vi "read_config.vi"() -> ()   [LabVIEW 2015]
uses:
  <vilib>/Utility/config.llb/Read Key (String).vi
  global/tcp_conn.vi
  global_config.vi
  <vilib>/Utility/config.llb/NI_LVConfig.lvlib
panel:
  out "服务器IP地址":string
  out "配置信息输出":T1
  out "默认上传数据输出":string[](array[string])
  out "value":string caption="data"
  out "info":string[](array[string])
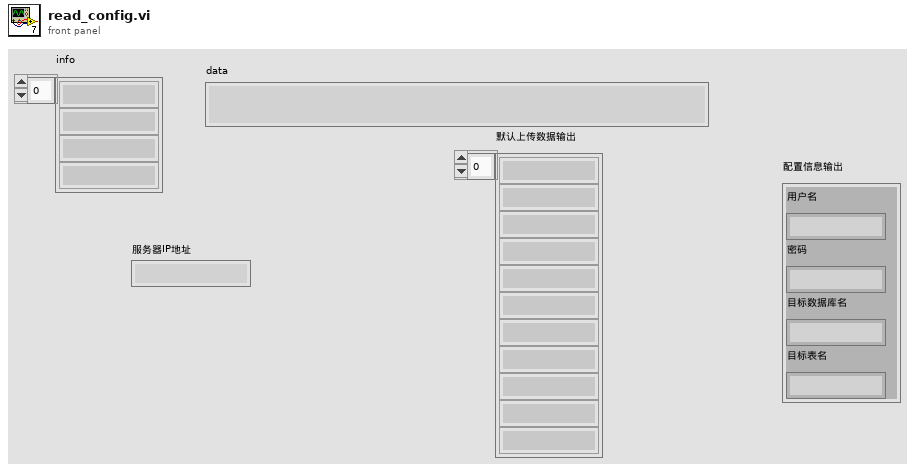
[diagram p1: front panel]
types:
  T1 = cluster{"用户名":string, "密码":string, "目标数据库名":string, "目标表名":string}
  T2 = enum32{"invalid app kind", "Development System", "Run Time System", "Student Edition", "Embedded LabVIEW", "Evaluation", "Custom"}
  T3 = typedef "NI_LVConfig.lvlib/Config Data RefNum.ctl" = refnum<k1>
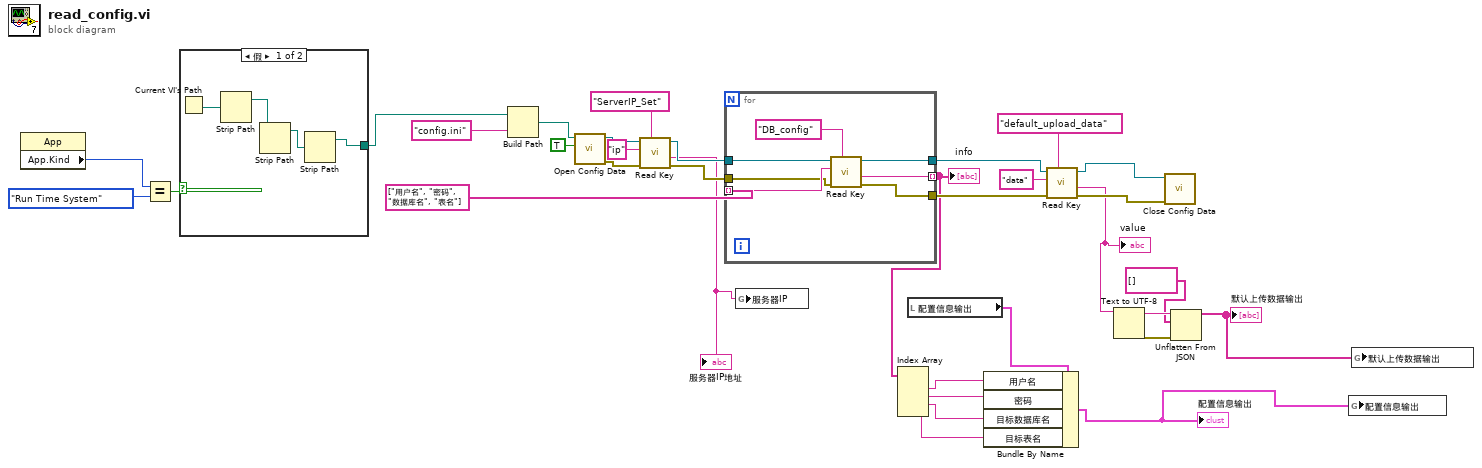
[diagram p0: block diagram]
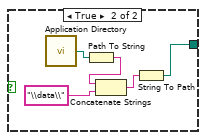
[diagram p2: hidden frame]
diagram:
  n1 = property class="App"() -> ("App.Kind"=w13:T2)  [unwired: 2 in, 2 out]
  n2 = Equal?(x=w13, y=T2."Run Time System" ("应用程序:类别")) -> (x = y?=w11:bool)
  n3 = case shown="假" w11 {
    tunnel: [w37 w39] -> w10
    frame False {
      n4 = Current VI's Path() -> (path=w34:path)
      n5 = Strip Path(path=w34) -> (stripped path=w35:path)  [unwired: 1 out]
      n6 = Strip Path(path=w35) -> (stripped path=w36:path)  [unwired: 1 out]
      n7 = Strip Path(path=w36) -> (stripped path=w37:path)  [unwired: 1 out]
    }
    frame True {
      n8 = call <vilib>:"Application Directory.vi"() -> ("Application Directory"=w42:path)
      n9 = Path To String(path=w42) -> (string=w41:string)
      n10 = Concatenate Strings(w41, "\\data\\" ("名称或相对路径")) -> (w38:string)
      n11 = String To Path(string=w38) -> (path=w39:path)
    }
  }
  n12 = Build Path(base path=w10, name or relative path="config.ini") -> (appended path=w32:path)
  n13 = call <vilib>:"Open Config Data.vi"("create file if necessary (T)"=TRUE, "configuration file path"=w32) -> ("error out"=w6:errorcluster, "refnum"=w7:T3)  [unwired: 7 in, 1 out]
  n14 = call-poly <vilib>:"Read Key.vi"("section"="ServerIP_Set", "error in (no error)"=w6, "key"="ip", "refnum"=w7) -> ("error out"=w4:errorcluster, "value"=w1:string, "refnum out"=w5:T3)  [unwired: 4 in, 1 out]
  "服务器IP地址" <- w1
  n15 = for {
    tunnel: string[] ["用户名", "密码", "数据库名", "表名"] ("info_name") -> [w48] mode=indexing
    tunnel: w5 -> [w47]
    tunnel: w4 -> [w46]
    tunnel: [w45] -> w14 mode=indexing
    tunnel: [w44] -> w29
    tunnel: [w43] -> w28
    n16 = call-poly <vilib>:"Read Key.vi"("section"="DB_config", "error in (no error)"=w46, "key"=w48, "refnum"=w47) -> ("error out"=w43:errorcluster, "value"=w45:string, "refnum out"=w44:T3)  [unwired: 4 in, 1 out]
  }
  "info" <- w14
  n17 = global write "tcp_conn.vi" "服务器IP"(w1) -> ()
  n18 = Index Array(array=w14) -> (element #1=w18:string, element #2=w17:string, element #3=w16:string, element #4=w15:string)  [unwired: 4 in]
  n19 = local read "配置信息输出"() -> (w19:T1)
  n20 = Bundle By Name(cluster=w19, "用户名"=w18, "密码"=w17, "目标数据库名"=w16, "目标表名"=w15) -> (w8:T1)
  "配置信息输出" <- w8
  n21 = call-poly <vilib>:"Read Key.vi"("section"="default_upload_data", "error in (no error)"=w28, "key"="data", "refnum"=w29) -> ("error out"=w24:errorcluster, "value"=w23:string, "refnum out"=w25:T3)  [unwired: 4 in, 1 out]
  "value" <- w23
  n22 = Text to UTF-8(11:w23) -> (0:w21:errorcluster, 3:w22:string)  [unwired: 2 in]
  n23 = call <vilib>:"Close Config Data.vi"("error in (no error)"=w24, "refnum"=w25) -> ()  [unwired: 8 in, 2 out]
  n24 = Unflatten From JSON(JSON string=w22, type and defaults=string[] [], error in (no error)=w21) -> (value=w9:string[])  [unwired: 4 in, 1 out]
  "默认上传数据输出" <- w9
  n25 = global write "global_config.vi" "配置信息输出"(w8) -> ()
  n26 = global write "global_config.vi" "默认上传数据输出"(w9) -> ()
